vi "IVIS FRET_Compute Intensities Arrays.vi"(9 "Liver Intensities":T1[](array[typedef]), 10 "UB Intensities":T1[](array[typedef]), 11 "Time Axis":dbl[](array[numeric])) -> (3 "Intensities Arrays":cluster{"Time Axis":dbl[], "Array":dbl[]}[](array[cluster]))   [LabVIEW 2021]
uses:
  IVIS FRET_Frame Image Intensities.ctl
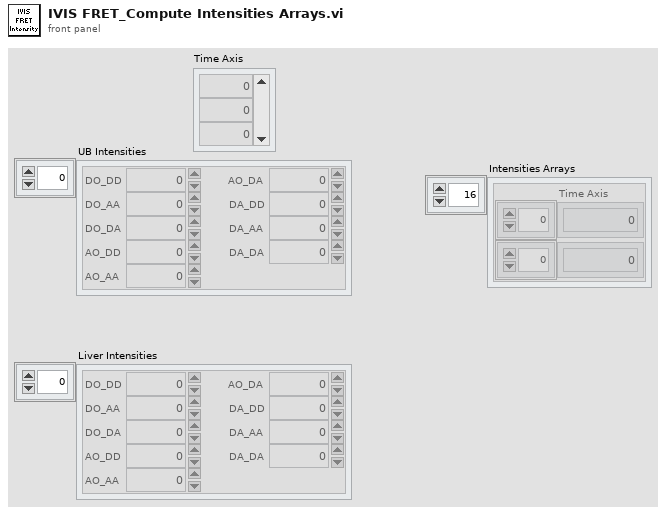
[diagram p1: front panel]
types:
  T1 = typedef "IVIS FRET_Frame Image Intensities.ctl" = cluster{"DO_DD":dbl, "DO_AA":dbl, "DO_DA":dbl, "AO_DD":dbl, "AO_AA":dbl, "AO_DA":dbl, "DA_DD":dbl, "DA_AA":dbl, "DA_DA":dbl}
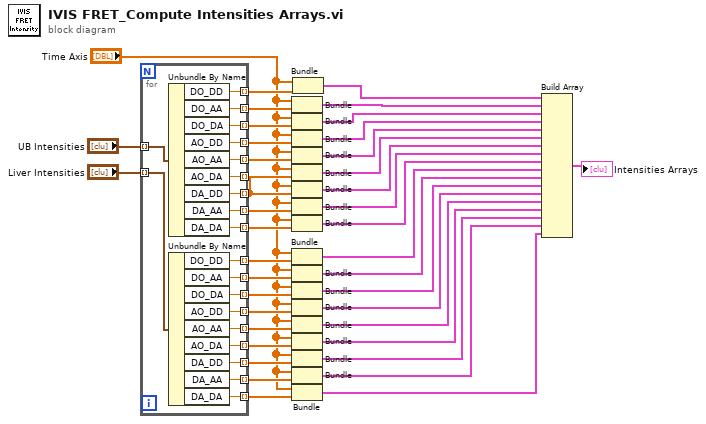
[diagram p0: block diagram]
diagram:
  n1 = for {
    tunnel: "UB Intensities" -> [w59] mode=indexing
    tunnel: "Liver Intensities" -> [w58] mode=indexing
    tunnel: [w57] -> w37 mode=indexing
    tunnel: [w56] -> w35 mode=indexing
    tunnel: [w55] -> w34 mode=indexing
    tunnel: [w54] -> w33 mode=indexing
    tunnel: [w53] -> _ mode=indexing
    tunnel: [w52] -> w32 mode=indexing
    tunnel: [w51] -> w31 mode=indexing
    tunnel: [w50] -> w30 mode=indexing
    tunnel: [w49] -> w29 mode=indexing
    tunnel: [w48] -> w28 mode=indexing
    tunnel: [w47] -> w27 mode=indexing
    tunnel: [w46] -> w26 mode=indexing
    tunnel: [w45] -> w25 mode=indexing
    tunnel: [w44] -> w24 mode=indexing
    tunnel: [w43] -> w23 mode=indexing
    tunnel: [w42] -> w22 mode=indexing
    tunnel: [w41] -> w21 mode=indexing
    tunnel: [w40] -> w3 mode=indexing
    n2 = Unbundle By Name(w59) -> ("DO_DD"=w40:dbl, "DO_AA"=w57:dbl, "DO_DA"=w56:dbl, "AO_DD"=w55:dbl, "AO_AA"=w54:dbl, "AO_DA"=w53:dbl, "DA_DD"=w52:dbl, "DA_AA"=w51:dbl, "DA_DA"=w50:dbl)
    n3 = Unbundle By Name(w58) -> ("DO_DD"=w49:dbl, "DO_AA"=w48:dbl, "DO_DA"=w47:dbl, "AO_DD"=w46:dbl, "AO_AA"=w45:dbl, "AO_DA"=w44:dbl, "DA_DD"=w43:dbl, "DA_AA"=w42:dbl, "DA_DA"=w41:dbl)
  }
  n4 = Bundle("Time Axis"="Time Axis", w37) -> (w36:cluster{"Time Axis":dbl[], dbl[]})  [unwired: 1 in]
  n5 = Bundle("Time Axis"="Time Axis", w35) -> (w20:cluster{"Time Axis":dbl[], dbl[]})  [unwired: 1 in]
  n6 = Bundle("Time Axis"="Time Axis", w34) -> (w19:cluster{"Time Axis":dbl[], dbl[]})  [unwired: 1 in]
  n7 = Bundle("Time Axis"="Time Axis", w33) -> (w18:cluster{"Time Axis":dbl[], dbl[]})  [unwired: 1 in]
  n8 = Bundle("Time Axis"="Time Axis", w32) -> (w17:cluster{"Time Axis":dbl[], dbl[]})  [unwired: 1 in]
  n9 = Bundle("Time Axis"="Time Axis", w32) -> (w16:cluster{"Time Axis":dbl[], dbl[]})  [unwired: 1 in]
  n10 = Bundle("Time Axis"="Time Axis", w31) -> (w15:cluster{"Time Axis":dbl[], dbl[]})  [unwired: 1 in]
  n11 = Bundle("Time Axis"="Time Axis", w30) -> (w14:cluster{"Time Axis":dbl[], dbl[]})  [unwired: 1 in]
  n12 = Bundle("Time Axis"="Time Axis", w29) -> (w13:cluster{"Time Axis":dbl[], dbl[]})  [unwired: 1 in]
  n13 = Bundle("Time Axis"="Time Axis", w28) -> (w12:cluster{"Time Axis":dbl[], dbl[]})  [unwired: 1 in]
  n14 = Bundle("Time Axis"="Time Axis", w27) -> (w11:cluster{"Time Axis":dbl[], dbl[]})  [unwired: 1 in]
  n15 = Bundle("Time Axis"="Time Axis", w26) -> (w10:cluster{"Time Axis":dbl[], dbl[]})  [unwired: 1 in]
  n16 = Bundle("Time Axis"="Time Axis", w25) -> (w9:cluster{"Time Axis":dbl[], dbl[]})  [unwired: 1 in]
  n17 = Bundle("Time Axis"="Time Axis", w24) -> (w8:cluster{"Time Axis":dbl[], dbl[]})  [unwired: 1 in]
  n18 = Bundle("Time Axis"="Time Axis", w23) -> (w7:cluster{"Time Axis":dbl[], dbl[]})  [unwired: 1 in]
  n19 = Bundle("Time Axis"="Time Axis", w22) -> (w6:cluster{"Time Axis":dbl[], dbl[]})  [unwired: 1 in]
  n20 = Bundle("Time Axis"="Time Axis", w21) -> (w5:cluster{"Time Axis":dbl[], dbl[]})  [unwired: 1 in]
  n21 = Bundle("Time Axis"="Time Axis", w3) -> (w1:cluster{"Time Axis":dbl[], dbl[]})  [unwired: 1 in]
  n22 = Build Array(w1, w36, w20, w19, w18, w17, w16, w15, w14, w13, w12, w11, w10, w9, w8, w7, w6, w5) -> (→"Intensities Arrays":cluster{"Time Axis":dbl[], dbl[]}[])
